vi "3-8 Case Structure.vi"() -> ()   [LabVIEW 2015]
doc: "This simple VI thorws a warning if the Current temp input is greater than the max temp input or less than the min temp input."
panel:
  out "Warning?":bool
  out "Warning Text":string
  in  "Max Temp":dbl=30.0
  in  "Min Temp":dbl=10.0
  in  "Current Temp":dbl=25.0
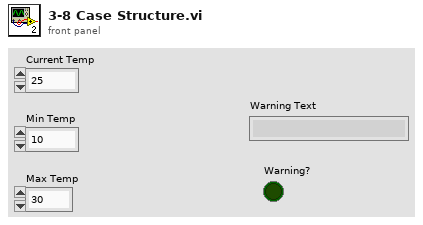
[diagram p1: front panel]
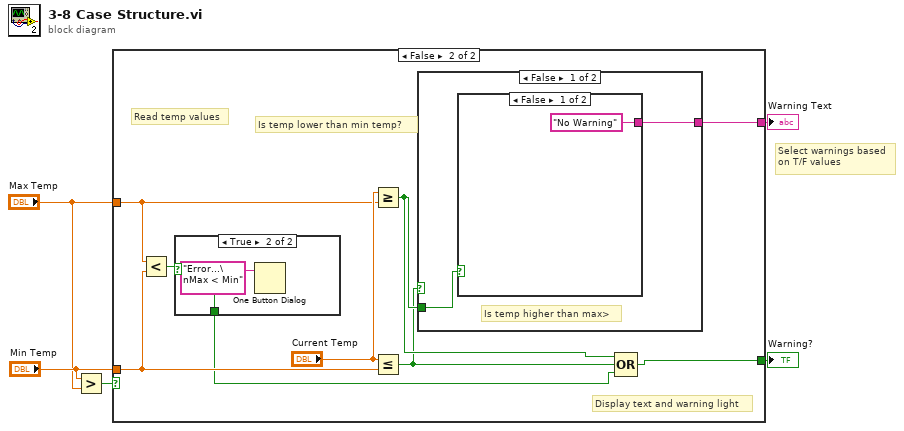
[diagram p0: block diagram]
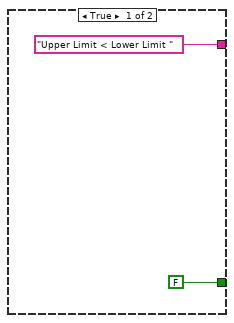
[diagram p2: hidden frame]
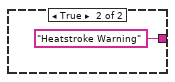
[diagram p4: hidden frame]
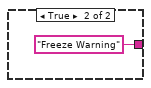
[diagram p5: hidden frame]
diagram:
  # "Select warnings based\non T/F values"
  n1 = Greater?(x="Min Temp", y="Max Temp") -> (0:w1:bool)
  n2 = case shown="False" w1 {
    tunnel: "Max Temp" -> [_ w14]
    tunnel: "Min Temp" -> [_ w12]
    tunnel: ["Upper Limit < Lower Limit " w15] -> w5
    tunnel: [FALSE w8] -> w4
    frame True {
    }
    frame False {
      # "Display text and warning light"
      # "Read temp values"
      # "Is temp lower than min temp?"
      n3 = Less?(x=w14, y=w12) -> (x < y?=w13:bool)
      n4 = case shown="True" w13 {
        selector: w13 -> [w17 w19]
        tunnel: [w17 w19] -> w9
        frame False {
        }
        frame True {
          n5 = One Button Dialog(message="Error...\nMax < Min") -> ()  [unwired: 1 in, 1 out]
        }
      }
      n6 = Greater Or Equal?(x="Current Temp", y=w14) -> (x >= y?=w11:bool)
      n7 = Less Or Equal?(x="Current Temp", y=w12) -> (x <= y?=w10:bool)
      n8 = case shown="False" w10 {
        tunnel: [w20 "Freeze Warning"] -> w15
        tunnel: w11 -> [w21 _]
        frame False {
          # "Is temp higher than max>"
          n9 = case shown="False" w21 {
            tunnel: ["No Warning" "Heatstroke Warning"] -> w20
            frame False {
            }
            frame True {
            }
          }
        }
        frame True {
        }
      }
      n10 = Compound Arithmetic op=OR(w11, w10, w9) -> (w8:bool)
    }
  }
  "Warning Text" <- w5
  "Warning?" <- w4
